vi "WriteChunk.vi"(3 "error in (no error)":errorcluster, 4 "data in":string, 5 "connection ID":refnum<k5>) -> (0 "error out":errorcluster, 1 "bytes written":i32, 2 "connection ID out":refnum<k5>)   [LabVIEW 2012]
panel:
  in  "Num Retries":i32=10
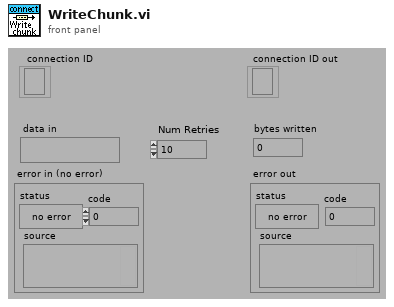
[diagram p1: front panel]
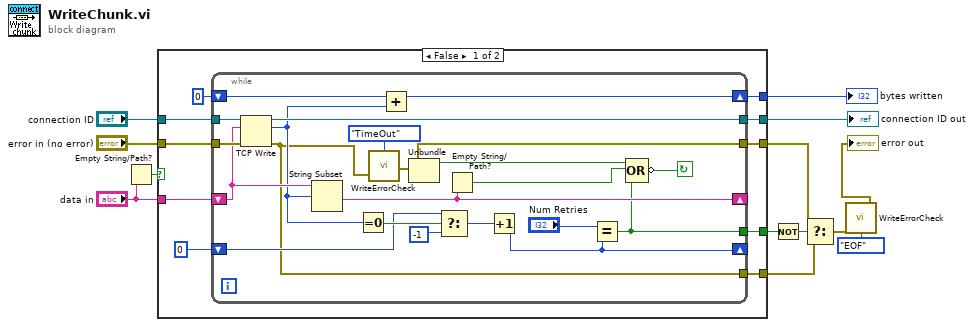
[diagram p0: block diagram]
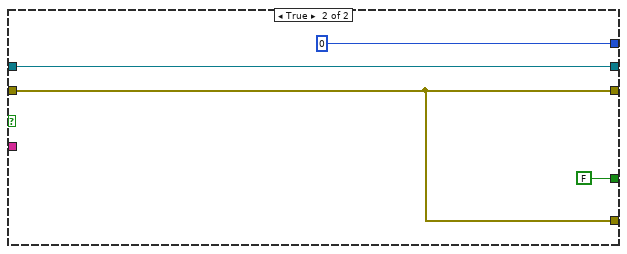
[diagram p2: hidden frame]
diagram:
  n1 = Empty String/Path?(string/path="data in") -> (empty?=w9:bool)
  n2 = case shown="False" w9 {
    tunnel: "data in" -> [w23 _]
    tunnel: [w22 0 ("y")] -> w7
    tunnel: [w20 w48] -> w6
    tunnel: [w19 w45] -> w13
    tunnel: "error in (no error)" -> [w18 w45]
    tunnel: "connection ID" -> [w17 w48]
    tunnel: [w15 FALSE] -> w11
    tunnel: [w14 w45] -> w12
    frame False {
      n3 = while {
        shift-left: 0 ("y") -> [w39]
        shift-right: [w38] -> w22
        tunnel: [w41] -> w20
        tunnel: [w24] -> w19
        shift-left: w23 -> [w42]
        shift-right: [w40] -> _
        tunnel: w18 -> [w43]
        tunnel: w17 -> [w44]
        shift-right: [w32] -> _
        shift-left: 0 -> [w34]
        tunnel: [w27] -> w15
        tunnel: [w26] -> w14
        stop <- w28 continue-if-true
        n4 = TCP Write(connection ID=w44, data in=w42, error in (no error)=w43) -> (connection ID out=w41:refnum<k5>, bytes written=w37:i32, error out=w26:errorcluster)  [unwired: 1 out]
        n5 = String Subset(string=w42, offset (0)=w37) -> (substring=w40:string)  [unwired: 1 out]
        n6 = Equal To 0?(x=w37) -> (x = 0?=w36:bool)
        n7 = call <userlib>:"WriteErrorCheck.vi"("error in (no error)"=w26, "Err Check"=enum16{"TimeOut", "EOF"}."TimeOut") -> ("error out"=w24:errorcluster)
        n8 = Add(x=w39, y=w37) -> (x+y=w38:i32)
        n9 = Unbundle(w24) -> ("status"=w30:bool)  [unwired: 2 out]
        n10 = Select(t=w34, s=w36, f=-1) -> (s? t:f=w33:i32)
        n11 = Empty String/Path?(string/path=w40) -> (empty?=w29:bool)
        n12 = Increment(x=w33) -> (x+1=w32:i32)
        n13 = Equal?(x="Num Retries", y=w32) -> (x = y?=w27:bool)
        n14 = Compound Arithmetic op=OR(w30, w29, w27) -> (invert w28:bool)
      }
    }
    frame True {
    }
  }
  "connection ID out" <- w6
  "bytes written" <- w7
  n15 = Not(x=w11) -> (.not. x?=w10:bool)
  n16 = Select(t=w13, s=w10, f=w12) -> (s? t:f=w2:errorcluster)
  n17 = call <userlib>:"WriteErrorCheck.vi"("error in (no error)"=w2, "Err Check"=enum16{"TimeOut", "EOF"}."EOF") -> ("error out"=→"error out":errorcluster)
